vi "Exponential Fit (LAR).vi"(0 "Y":dbl[](array[numeric]), 5 "X":dbl[](array[numeric]), 7 "Weight":dbl[](array[numeric]), 9 "tolerance":dbl=-1.0 format="%#_3g", 11 "Initial Coefficients":dbl[](array[numeric]), 12 "algorithm":u16(ring) items=["Semi-Log", "Iterative"]) -> (4 "Best Exponential Fit":dbl[](array[numeric]), 6 "amplitude":dbl, 8 "damping":dbl, 14 "residue":dbl, 15 "error":i32)   [LabVIEW 2017, in "NI_AALPro.lvlib"]
uses:
  NI_AALPro.lvlib
  <resource>/lvanlys.dll
panel:
  # "LAR Exponential Fit"
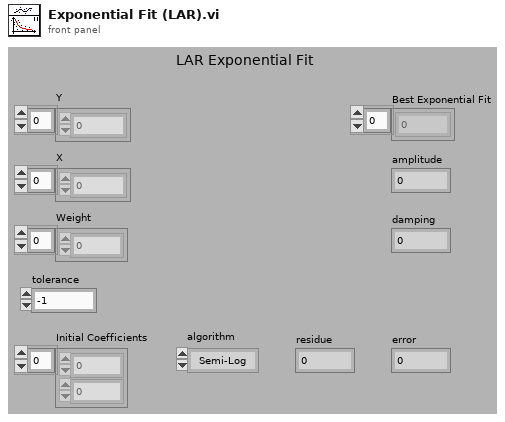
[diagram p1: front panel]
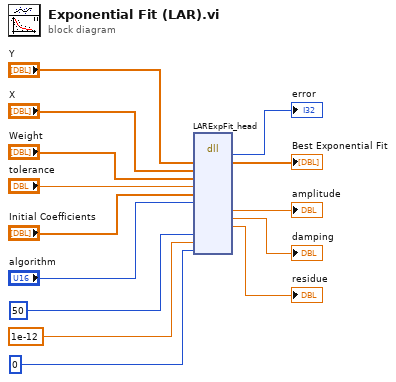
[diagram p0: block diagram]
diagram:
  n1 = dll-call lib="C:/Program Files (x86)/National Instruments/LabVIEW 2017/resource/lvanlys.*" fn="LARExpFit_head"("y"="Y", "x"="X", "weight"="Weight", "tolerance"="tolerance", "intial coef"="Initial Coefficients", "algorithm"="algorithm", "maxIter"=50, "absTol"=1e-12, "isCoef"=0 ("maxIter")) -> (→"error":i32, "y"=→"Best Exponential Fit":dbl[], "amp"=→"amplitude":dbl, "damping"=→"damping":dbl, "mearErr"=→"residue":dbl)  [unwired: 14 in, 2 out]
